vi "Trajectory Adaptation Algorithm_v3.vi"(0 "start (xi,yi)":dbl[](array[numeric])=[0.0, 5.0] format="%.2f", 1 "baseline (x,y,z)":dbl[](array[numeric])=[0.0, 5.0, 0.0] format="%.2f", 3 "z_assign":dbl, 5 "(r_eye,r_assign)":dbl[](array[numeric])=[5.0, 1.0], 7 "Tassign":dbl[](array[numeric])=[0.0, 5.0], 9 "Tt":dbl, 11 "Th":dbl, 12 "index":i32) -> (4 "rerouted (x,y,z)":dbl[](array[numeric])=[0.0, 5.0, 0.0])   [LabVIEW 2010]
doc: "This VI transforms the current (x,y) into a new location based on the assigned radius R assign and assigned translation vector Tassign. The location is index/time dependent: the frist Tt seconds, rotation matrix and translation vector ramp up linearly, and then it would stay for another Th seconds, after that they ramp down to what they originally were and stay there unless otherwise told to.\n\nInterrupt is possible because of the additional registers added, namely, the new adaptation can be demanded while the previos one hasn't finished yet."
uses:
  <vilib>/Analysis/NI_AALBase.lvlib
  <vilib>/Analysis/baseanly.llb/A x Vector.vi
  <vilib>/Analysis/Matrix/NI_Matrix.lvlib
  <vilib>/Analysis/Matrix/Numeric/Conversions/Array To Matrix - RA2.vi
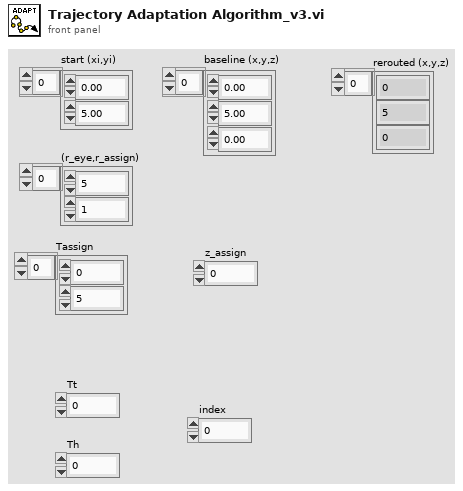
[diagram p1: front panel]
types:
  T1 = typedef "NI_Matrix.lvlib/RealMatrix.ctl" = dbl[][]
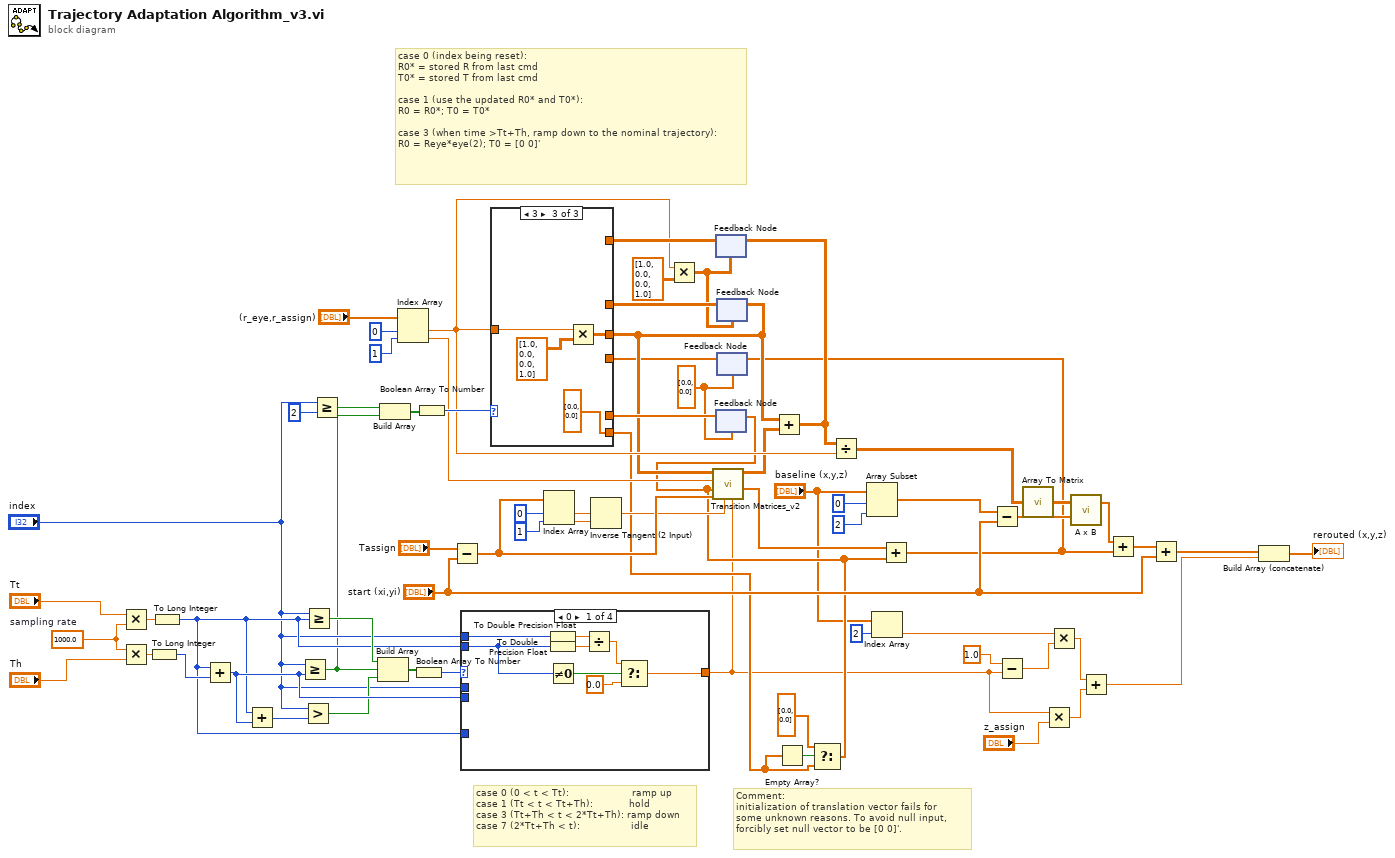
[diagram p0: block diagram]
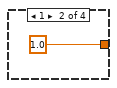
[diagram p4: hidden frame]
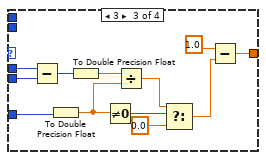
[diagram p5: hidden frame]
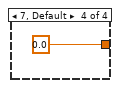
[diagram p6: hidden frame]
diagram:
  w18 = dbl[] [0.0, 0.0] ("Assign Point")
  w65 = 1000.0  # sampling rate
  # "Comment:\ninitialization of translation vector fails for\nsome unknown reasons. To avoid null input,\nforcibly set null vector to be [0 0]'."
  # "case 0 (index being reset):\nR0* = stored R from last cmd\nT0* = stored T from last cmd\n\ncase 1 (use the updated R0* and T0*):\nR0 = R0*; T0 = T0*\n\ncase 3 (when time >Tt+Th, ramp down to the nominal trajectory):\nR0 = Reye*eye(2); T0 = [0 0]'"
  # "case 0 (0 < t < Tt):                     ramp up\ncase 1 (Tt < t < Tt+Th):            hold\ncase 3 (Tt+Th < t < 2*Tt+Th): ramp down\ncase 7 (2*Tt+Th < t):                 idle"
  n1 = Multiply(x="Tt", y=w65) -> (x*y=w67:dbl)
  n2 = Multiply(x=w65, y="Th") -> (x*y=w68:dbl)
  n3 = To Long Integer(number=w68) -> (32bit integer=w66:i32)
  n4 = To Long Integer(number=w67) -> (32bit integer=w46:i32)
  n5 = Add(x=w46, y=w66) -> (x+y=w47:i32)
  n6 = Add(x=w46, y=w47) -> (x+y=w61:i32)
  n7 = Greater Or Equal?(x="index", y=w47) -> (x >= y?=w28:bool)
  n8 = Greater?(x="index", y=w61) -> (0:w44:bool)
  n9 = Greater Or Equal?(x="index", y=w46) -> (x >= y?=w64:bool)
  n10 = Greater Or Equal?(x="index", y=2) -> (x >= y?=w32:bool)
  n11 = Build Array(w64, w28, w44) -> (w63:bool[])
  n12 = Build Array(w32, w28) -> (w43:bool[])
  n13 = Index Array(array="(r_eye,r_assign)", index #1=0 ("index"), index #2=1 ("index")) -> (element #1=w34:dbl, element #2=w39:dbl)
  n14 = Boolean Array To Number(Boolean array=w63) -> (number=w62:u32)
  n15 = Boolean Array To Number(Boolean array=w43) -> (number=w42:u32)
  n16 = Subtract(x="Tassign", y="start (xi,yi)") -> (x-y=w51:dbl[])
  n17 = case shown="0" w62 {
    tunnel: w46 -> [w73 _ _ _]
    tunnel: "index" -> [w74 _ _ _]
    tunnel: [w70 1.0 w86 0.0] -> w12
    tunnel: "index" -> [_ _ w88 _]
    tunnel: w47 -> [_ _ w87 _]
    tunnel: w46 -> [_ _ w83 _]
    frame 0 {
      n18 = To Double Precision Float(number=w74) -> (double precision float=w76:dbl)
      n19 = To Double Precision Float(number=w73) -> (double precision float=w75:dbl)
      n20 = Not Equal To 0?(x=w73) -> (x != 0?=w72:bool)
      n21 = Divide(x=w76, y=w75) -> (x/y=w71:dbl)
      n22 = Select(t=w71, s=w72, f=0.0) -> (s? t:f=w70:dbl)
    }
    frame 1 {
    }
    frame 3 {
      n23 = Subtract(x=w88, y=w87) -> (x-y=w85:i32)
      n24 = To Double Precision Float(number=w83) -> (double precision float=w80:dbl)
      n25 = To Double Precision Float(number=w85) -> (double precision float=w84:dbl)
      n26 = Not Equal To 0?(x=w80) -> (x != 0?=w82:bool)
      n27 = Divide(x=w84, y=w80) -> (x/y=w78:dbl)
      n28 = Select(t=w78, s=w82, f=0.0) -> (s? t:f=w79:dbl)
      n29 = Subtract(x=1.0, y=w79) -> (x-y=w86:dbl)
    }
    frame 7, Default {
    }
  }
  n30 = Index Array(array=w51, index #1=0 ("index"), index #2=1 ("index")) -> (element #1=w57:dbl, element #2=w56:dbl)
  n31 = Inverse Tangent (2 Input)(1:w56, 2:w57) -> (0:w37:dbl)
  n32 = Multiply(x=w34, y=dbl[][] [[1.0, 0.0], [0.0, 1.0]]) -> (x*y=w30:dbl[][])
  n33 = feedback #1(w30) -> (w38:dbl[][])
  n34 = feedback #2(w18) -> (w29:dbl[])
  n35 = feedback #3(w30) -> (w31:dbl[][])
  n36 = feedback #4(w18) -> (w21:dbl[])
  n37 = case shown="3" w42 {
    tunnel: w34 -> [_ _ w97]
    tunnel: [w92 w94 w96] -> w25
    tunnel: w38 -> [w92 _ _]
    tunnel: w21 -> [w91 _ _]
    tunnel: [w91 w93 dbl[] [0.0, 0.0]] -> w17
    tunnel: w31 -> [_ w94 _]
    tunnel: w29 -> [_ w93 _]
    frame 0, Default {
    }
    frame 1 {
    }
    frame 3 {
      n38 = Multiply(x=w97, y=dbl[][] [[1.0, 0.0], [0.0, 1.0]]) -> (x*y=w96:dbl[][])
    }
  }
  n39 = feedback-in #3(w25) -> ()
  n40 = Empty Array?(array=w17) -> (empty?=w20:bool)
  n41 = Select(t=dbl[] [0.0, 0.0], s=w20, f=w17) -> (s? t:f=w16:dbl[])
  n42 = call "Transition Matrices_v2.vi"("alpha"=w12, "theta"=w37, "Tassign"=w51, "T0"=w16, "Rassign"=w39, "R0"=w25) -> ("Translation Vector"=w23:dbl[], "Rotation Matrix"=w24:dbl[][])  [unwired: 4 in]
  n43 = feedback-in #2(w16) -> ()
  n44 = Add(x=w25, y=w24) -> (x+y=w33:dbl[][])
  n45 = feedback-in #1(w33) -> ()
  n46 = Divide(x=w33, y=w34) -> (x/y=w41:dbl[][])
  n47 = Array Subset(array="baseline (x,y,z)", index=0, length=2) -> (w6:dbl[])
  n48 = Index Array(array="baseline (x,y,z)", index=2) -> (element=w3:dbl)
  n49 = Add(x=w23, y=w16) -> (x+y=w22:dbl[])
  n50 = feedback-in #4(w22) -> ()
  n51 = Subtract(x=w6, y="start (xi,yi)") -> (x-y=w54:dbl[])
  n52 = Subtract(x=1.0, y=w12) -> (x-y=w14:dbl)
  n53 = call-poly <vilib>:"Array To Matrix.vi"("Real 2D Array"=w41) -> ("Real Matrix"=w55:T1)
  n54 = Multiply(x=w12, y="z_assign") -> (x*y=w10:dbl)
  n55 = Multiply(x=w3, y=w14) -> (x*y=w11:dbl)
  n56 = call-poly <vilib>:"A x B.vi"("Vector"=w54, "A"=w55) -> ("A x Vector"=w60:dbl[])  [unwired: 1 out]
  n57 = Add(x=w11, y=w10) -> (x+y=w7:dbl)
  n58 = Add(x=w60, y=w22) -> (x+y=w53:dbl[])
  n59 = Add(x=w53, y="start (xi,yi)") -> (x+y=w9:dbl[])
  n60 = Build Array (concatenate)(w9, w7) -> (→"rerouted (x,y,z)":dbl[])
